vi "Passing Paramters String.vi"(8 "error in (no error)":errorcluster, 11 "str":string) -> (0 "error out":errorcluster, 2 "function return":i32, 3 "str out":string)   [LabVIEW 2009, in "LabVIEWWrapper_PassingDataSampleDLL.lvlib"]
doc: "int PassingParamters_String (char *str);"
uses:
  LabVIEWWrapper_PassingDataSampleDLL.lvlib
  PassingDataSampleDLL.dll
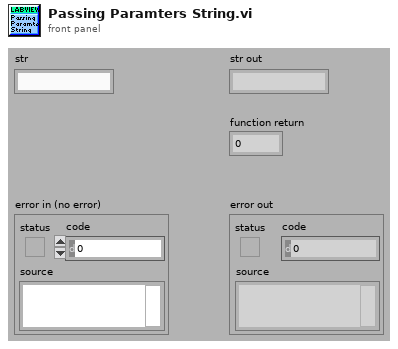
[diagram p1: front panel]
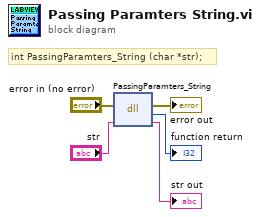
[diagram p0: block diagram]
diagram:
  # "int PassingParamters_String (char *str);"
  n1 = dll-call lib="C:/My Dropbox/Systems Engineering Application/SDK/C Integration/LabVIEWWrapper/PassingDataSampleDLL.*" fn="PassingParamters_String"(error in="error in (no error)", "str"="str") -> (error out=→"error out":errorcluster, →"function return":i32, "str"=→"str out":string)  [unwired: 2 in, 1 out]
